vi "FGVAuto.vi"(10 "Motor Distance In":dbl, 11 "Mode":enum16{"Initializing", "Setting", "Reading"}(ring)) -> (3 "Motor Distance Out":dbl)   [LabVIEW 2017]
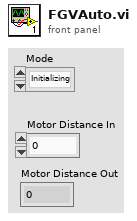
[diagram p1: front panel]
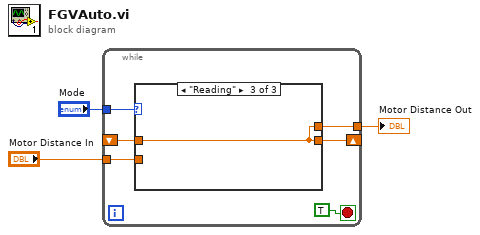
[diagram p0: block diagram]
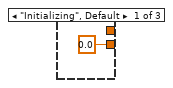
[diagram p2: hidden frame]
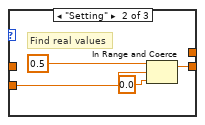
[diagram p3: hidden frame]
diagram:
  n1 = while {
    shift-right: [w8] -> _
    shift-left: _ -> [w6]
    tunnel: "Mode" -> [w9]
    tunnel: "Motor Distance In" -> [w5]
    tunnel: [w4] -> w1
    stop <- TRUE stop-if-true
    n2 = case shown="\"Reading\"" w9 {
      tunnel: [0.0 w11 w15] -> w8
      tunnel: w6 -> [_ _ w15]
      tunnel: w5 -> [_ w14 _]
      tunnel: [_ _ w15] -> w4
      frame "Initializing", Default {
      }
      frame "Setting" {
        # "Find real values"
        n3 = In Range and Coerce(upper limit=0.5, x=w14, lower limit=0.0) -> (coerced(x)=w11:dbl)  [unwired: 1 out]
      }
      frame "Reading" {
      }
    }
  }
  "Motor Distance Out" <- w1
